vi "Write starting address.vi"(8 "error in":errorcluster, 10 "starting address":u16, 11 "Modbus Module Channel in":refnum<class "Modbus Module Channel.lvclass">) -> (0 "error out":errorcluster, 3 "Modbus Module Channel out":refnum<class "Modbus Module Channel.lvclass">)   [LabVIEW 2013, in "Modbus Module Channel.lvclass"]
uses:
  Modbus Module Channel.lvclass
  Modbus Module Channel.lvclass/Modbus Module Channel.ctl
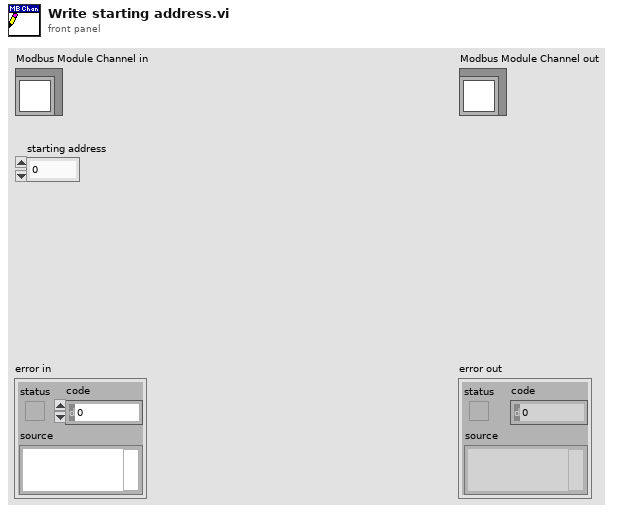
[diagram p1: front panel]
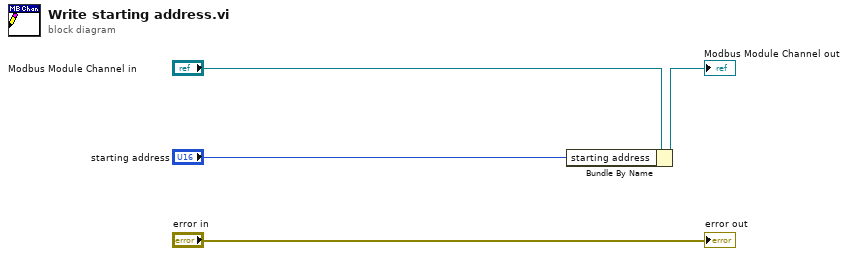
[diagram p0: block diagram]
diagram:
  n1 = Bundle By Name(cluster="Modbus Module Channel in", "starting address"="starting address") -> (→"Modbus Module Channel out":refnum<class "Modbus Module Channel.lvclass">)
  "error out" <- "error in"
